vi "FPGA.vi"(7 "LabVIEW Web Service Request":refnum<class "Web Request.lvclass">, 9 "RP_SaveData":dbl, 10 "RP_Stop":dbl, 11 "RP_Start":dbl) -> (1 "Chassis Temperature":dbl, 2 "value":string)   [LabVIEW 2020]
uses:
  <vilib>/wsapi/Web Request.lvclass
panel:
  # "Use the Web Service Request input terminal to call the VIs on the Web Services palette. Do not remove it from the connector pane unless you don't need access to the palette."
  # "Each additional control wired to the connector pane will be available as an input in the URL. To include an indicator in terminal-mode output (the default setting), it must also be wired to the connector pane."
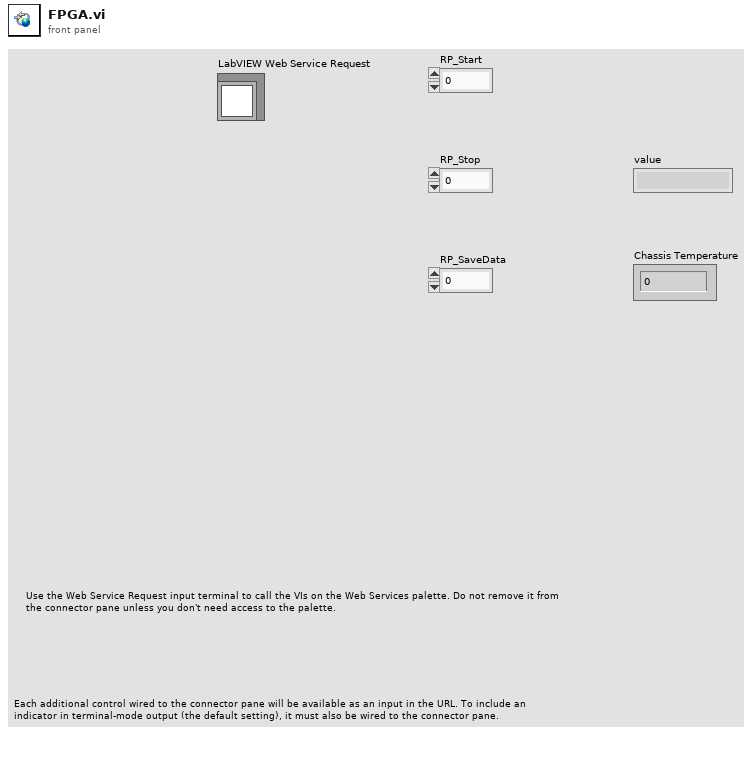
[diagram p1: front panel]
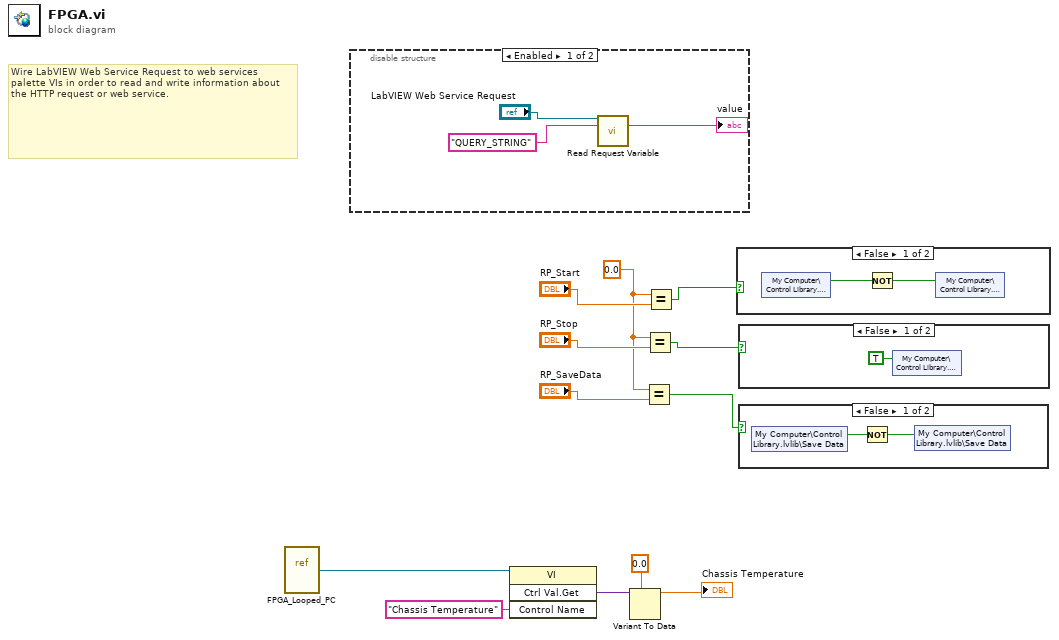
[diagram p0: block diagram]
diagram:
  w4 = 0.0 ("x")
  # "Wire LabVIEW Web Service Request to web services palette VIs in order to read and write information about the HTTP request or web service."
  n1 = vi-ref "FPGA_Looped_PC.vi"() -> (w11:refnum<vi>)
  n2 = disable-structure shown="Enabled" {
    frame Enabled {
      n3 = call <vilib>:"Read Request Variable.vi"("LabVIEW Web Service Request"="LabVIEW Web Service Request", "variable name"="QUERY_STRING") -> ("value"=→"value":string)  [unwired: 11 in, 2 out]
    }
    frame Disabled {
    }
  }
  n4 = invoke class="VI" method="Ctrl Val.Get"(reference=w11, "Control Name"="Chassis Temperature") -> ("Get Control Value Variant"=w10:variant)  [unwired: 2 in, 3 out]
  n5 = Variant To Data(type=0.0, Variant=w10) -> (data=→"Chassis Temperature":dbl)  [unwired: 1 in, 1 out]
  n6 = Equal?(x=w4, y="RP_SaveData") -> (x = y?=w2:bool)
  n7 = Equal?(x=w4, y="RP_Stop") -> (x = y?=w1:bool)
  n8 = Equal?(x=w4, y="RP_Start") -> (x = y?=w3:bool)
  n9 = case shown="False" w3 {
    frame False {
      n10 = shared-variable "My Computer\\Control Library.lvlib\\Start"() -> (w17:bool)  [unwired: 1 in, 1 out]
      n11 = Not(x=w17) -> (.not. x?=w16:bool)
      n12 = shared-variable "My Computer\\Control Library.lvlib\\Start"(w16) -> ()  [unwired: 1 in, 1 out]
    }
    frame True {
    }
  }
  n13 = case shown="False" w1 {
    frame False {
      n14 = shared-variable "My Computer\\Control Library.lvlib\\Stop"(TRUE ("Stop")) -> ()  [unwired: 1 in, 1 out]
    }
    frame True {
    }
  }
  n15 = case shown="False" w2 {
    frame False {
      n16 = shared-variable "My Computer\\Control Library.lvlib\\Save Data"() -> (w20:bool)  [unwired: 1 in, 1 out]
      n17 = Not(x=w20) -> (.not. x?=w19:bool)
      n18 = shared-variable "My Computer\\Control Library.lvlib\\Save Data"(w19) -> ()  [unwired: 1 in, 1 out]
    }
    frame True {
    }
  }
